vi "getBufferQuantity.vi"(8 "error in (no error)":errorcluster, 11 "Electrometer in":refnum<class "Electrometer.lvclass">) -> (0 "error out":errorcluster, 2 "quant":i32, 3 "Electrometer out":refnum<class "Electrometer.lvclass">)   [LabVIEW 2016, in "Electrometer.lvclass"]
uses:
  Electrometer.lvclass
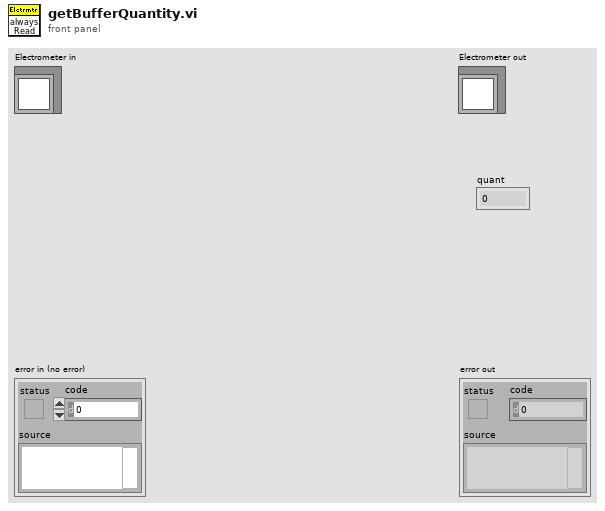
[diagram p1: front panel]
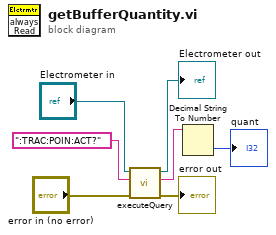
[diagram p0: block diagram]
diagram:
  n1 = call "executeQuery.vi"("error in (no error)"="error in (no error)", "command"=":TRAC:POIN:ACT?", "Electrometer in"="Electrometer in") -> ("error out"=→"error out":errorcluster, "result"=w3:string, "Electrometer out"=→"Electrometer out":refnum<class "Electrometer.lvclass">)  [unwired: 6 in]
  n2 = Decimal String To Number(string=w3) -> (number=→"quant":i32)  [unwired: 2 in, 1 out]
